vi "PointerArray_Offset.vi"(7 "Buffer":T1, 10 "Total Starting Offset":i32, 11 "Pointer Array":refnum<class "_Pointer.lvclass">[](array[class])) -> (3 "Pointer Array Out":refnum<class "_Pointer.lvclass">[](array[class]))   [LabVIEW 2020, in "WavBuf.lvclass"]
uses:
  WavBuf/WavBuf.lvclass
  Pointer/_Pointer.lvclass
  TypeDefs_Utility/Ref_DVR_Buffer.ctl
  Universal Controls/Waveform_Data.ctl
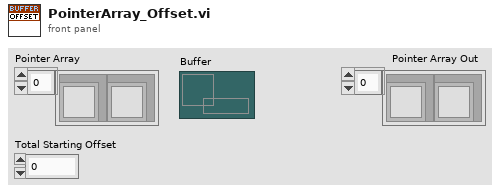
[diagram p1: front panel]
types:
  T1 = typedef "Ref_DVR_Buffer.ctl" = refnum<data-value>
  T2 = typedef "Waveform_Data.ctl" = waveform(dbl)
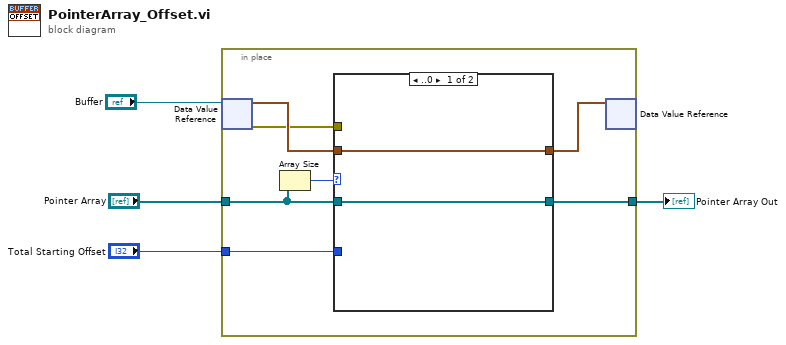
[diagram p0: block diagram]
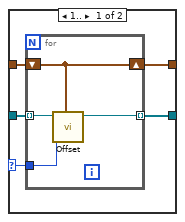
[diagram p3: hidden frame]
diagram:
  n1 = in-place {
    in-place-border: [w11] -> w4
    in-place-border: "Total Starting Offset" -> [w10]
    in-place-border: "Pointer Array" -> [w9]
    n2 = in-place-dvr #1("Buffer") -> (w7:T2, w5:errorcluster)
    n3 = Array Size(array=w9) -> (size(s)=w8:i32)
    n4 = case shown="..0" w8 {
      tunnel: [w13 w18] -> w11
      tunnel: w10 -> [_ w17]
      tunnel: w9 -> [w13 w16]
      tunnel: w7 -> [w12 w15]
      tunnel: [w12 w14] -> w6
      tunnel: w5 -> [_ _]
      frame ..0 {
      }
      frame 1.. {
        n5 = case shown="..0" w17 {
          selector: w17 -> [w23 _]
          tunnel: w16 -> [w22 w29]
          tunnel: [w21 w29] -> w18
          tunnel: w15 -> [w20 w28]
          tunnel: [w19 w28] -> w14
          frame 1.. {
            n6 = for {
              tunnel: w23 -> [w25]
              tunnel: w22 -> [w27] mode=indexing
              tunnel: [w26] -> w21 mode=indexing
              shift-right: [w24] -> w19
              shift-left: w20 -> [w24]
              n7 = call-dynamic "Offset.vi"("Raw Data Waveform"=w24, "Offset"=w25, "((Pointer))"=w27) -> ("((Pointer)) Out"=w26:refnum<class "_Pointer.lvclass">)  [unwired: 8 in]
            }
          }
          frame ..0 {
          }
        }
      }
    }
    n8 = in-place-dvr #1(w6) -> ()  [unwired: 2 out]
  }
  "Pointer Array Out" <- w4
